vi "SRV_Evaluate Parsed Formula String.vi"(8 "error in (no error)":errorcluster, 9 "Parsed Formula":cluster{"Table":i32[][], "Y Values":dbl[]} {"Y Values" format="%.2f"}, 11 "Variable v":dbl) -> (0 "error out":errorcluster, 2 "Value out":dbl format="%0.2f")   [LabVIEW 2014]
doc: "Evaluates the previously parsed formula.\n\n\nAuthor: Mike Schultz (mschultz11711@gmail.com)"
uses:
  <vilib>/gmath/NI_Gmath.lvlib
panel:
  # "operator"
  # "register1"
  # "register2"
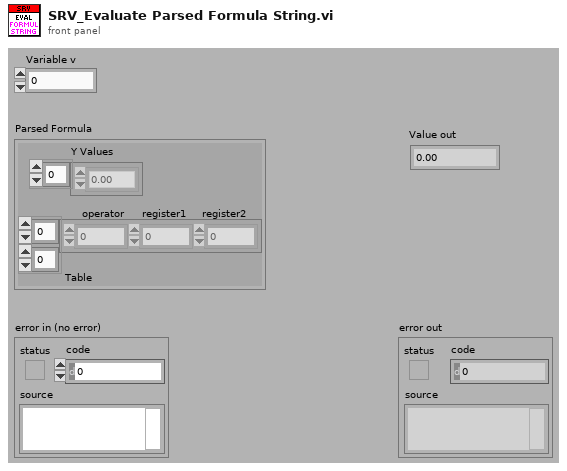
[diagram p1: front panel]
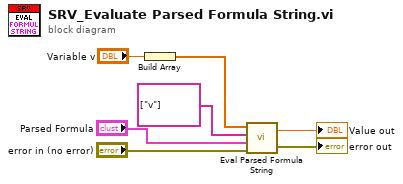
[diagram p0: block diagram]
diagram:
  n1 = Build Array("Variable v") -> (w5:dbl[])
  n2 = call <vilib>:"Eval Parsed Formula String.vi"("error in (no error)"="error in (no error)", "Parsed Formula"="Parsed Formula", "Variables"=string[] ["v"], "X Values"=w5) -> ("error out"=→"error out":errorcluster, "y value"=→"Value out":dbl)
